vi "Get User Data.vi"(10 "USER/ITEM DATA TRANSFER":T1(array[cluster]), 11 "REFERENCES":T2) -> (2 "USER/ITEM DATA TRANSFER OUT":T1(array[cluster]), 3 "REFERENCES OUT":T2)   [LabVIEW 2019]
uses:
  Controls/References Cluster.ctl
  Controls/Custom Calendar/Custom Calendar.xctl
  Controls/Table Data Types/User Data Type.ctl
  <vilib>/vision/Image Controls.llb/IMAQ Image.ctl
  <vilib>/addons/database/Connection.llb/DB Tools Open Connec (String).vi
  <vilib>/addons/database/_DB Variant To Data/Database Variant To Data.xnode
  <vilib>/addons/database/NI_Database_API.lvlib
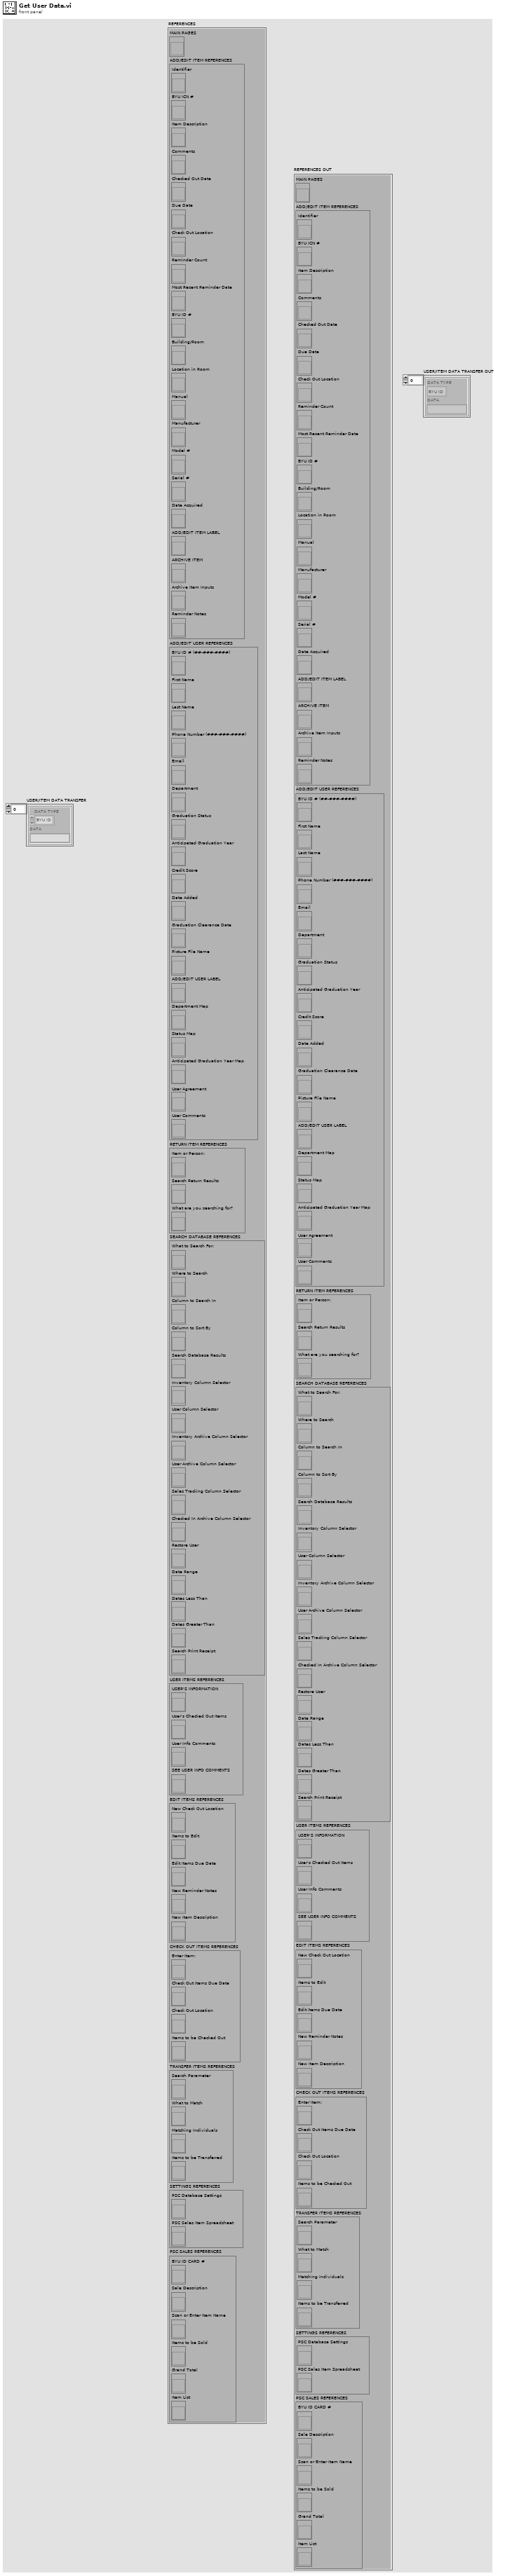
[diagram p1: front panel]
types:
  T1 = cluster{"DATA TYPE":enum16{"BYU ID", "ME#/IDENTIFIER", "BYU ICN"}, "DATA":string}[]
  T2 = typedef "References Cluster.ctl" = cluster{"MAIN PAGES":refnum<vi>, "ADD/EDIT ITEM REFERENCES":cluster{"Identifier":refnum<vi>, "BYU ICN #":refnum<vi>, "Item Description":refnum<vi>, "Comments":refnum<vi>, "Checked Out Date":refnum<vi>, "Due Date":refnum<vi>, "Check Out Location":refnum<vi>, "Reminder Count":refnum<vi>, "Most Recent Reminder Date":refnum<vi>, "BYU ID #":refnum<vi>, "Building/Room":refnum<vi>, "Location in Room":refnum<vi>, "Manual":refnum<vi>, "Manufacturer":refnum<vi>, "Model #":refnum<vi>, "Serial #":refnum<vi>, "Date Acquired":refnum<vi>, "ADD/EDIT ITEM LABEL":refnum<vi>, "ARCHIVE ITEM":refnum<vi>, "Archive Item Inputs":refnum<vi>, "Reminder Notes":refnum<vi>}, "ADD/EDIT USER REFERENCES":cluster{"BYU ID # (##-###-####)":refnum<vi>, "First Name":refnum<vi>, "Last Name":refnum<vi>, "Phone Number (###-###-####)":refnum<vi>, "Email":refnum<vi>, "Department":refnum<vi>, "Graduation Status":refnum<vi>, "Anticipated Graduation Year":refnum<vi>, "Credit Score":refnum<vi>, "Date Added":refnum<vi>, "Graduation Clearance Date":refnum<vi>, "Picture File Name":refnum<vi>, "ADD/EDIT USER LABEL":refnum<vi>, "Department Map":refnum<vi>, "Status Map":refnum<vi>, "Anticipated Graduation Year Map":refnum<vi>, "User Agreement":refnum<vi>, "User Comments":refnum<vi>}, "RETURN ITEM REFERENCES":cluster{"Item or Person:":refnum<vi>, "Search Return Results":refnum<vi>, "What are you searching for?":refnum<vi>}, "SEARCH DATABASE REFERENCES":cluster{"What to Search For:":refnum<vi>, "Where to Search":refnum<vi>, "Column to Search In":refnum<vi>, "Column to Sort By":refnum<vi>, "Search Database Results":refnum<vi>, "Inventory Column Selector":refnum<vi>, "User Column Selector":refnum<vi>, "Inventory Archive Column Selector":refnum<vi>, "User Archive Column Selector":refnum<vi>, "Sales Tracking Column Selector":refnum<vi>, "Checked In Archive Column Selector":refnum<vi>, "Restore User":refnum<vi>, "Date Range":refnum<vi>, "Dates Less Than":refnum<vi>, "Dates Greater Than":refnum<vi>, "Search Print Receipt":refnum<vi>}, "USER ITEMS REFERENCES":cluster{"USER'S INFORMATION":refnum<vi>, "User's Checked Out Items":refnum<vi>, "User Info Comments":refnum<vi>, "SEE USER INFO COMMENTS":refnum<vi>}, "EDIT ITEMS REFERENCES":cluster{"New Check Out Location":refnum<vi>, "Items to Edit":refnum<vi>, "Edit Items Due Date":refnum<vi>, "New Reminder Notes":refnum<vi>, "New Item Description":refnum<vi>}, "CHECK OUT ITEMS REFERENCES":cluster{"Enter Item:":refnum<vi>, "Check Out Items Due Date":refnum<vi>, "Check Out Location":refnum<vi>, "Items to be Checked Out":refnum<vi>}, "TRANSFER ITEMS REFERENCES":cluster{"Search Parameter":refnum<vi>, "What to Match":refnum<vi>, "Matching Individuals":refnum<vi>, "Items to be Transferred":refnum<vi>}, "SETTINGS REFERENCES":cluster{"PSC Database Settings":refnum<vi>, "PSC Sales Item Spreadsheet":refnum<vi>}, "PSC SALES REFERENCES":cluster{"BYU ID CARD #":refnum<vi>, "Sale Description":refnum<vi>, "Scan or Enter Item Name":refnum<vi>, "Items to be Sold":refnum<vi>, "Grand Total":refnum<vi>, "Item List":refnum<vi>}}
  T3 = enum32{"IDLE", "ADD/EDIT USER", "ADD/EDIT ITEM", "RETURN ITEMS", "SEARCH DATABASE", "USER ITEMS", "CHECK OUT ITEMS", "EDIT ITEMS", "TRANSFER ITEMS", "PSC SALES", "ATRIUM", "INVENTORY TRACKING", "SETTINGS"}
  T4 = typedef "IMAQ Image.ctl" = refnum<image>
  T5 = cluster{"BYU ID #":string, "First Name":string, "Last Name":string, "Phone Number":string, "Email":string, "Department":string, "Graduation Status":string, "Grad Year":string, "Credit Score":string, "Date Added":string, "Graduation Clearance Date":string, "User Items Photo":T4}
  T6 = typedef "User Data Type.ctl" = cluster{"BYU ID #":string, "First Name":string, "Last Name":string, "Phone Number":string, "Email":string, "Department":string, "Graduation Status":string, "Anticipated Graduation Year":string, "Credit Score":dbl, "Date Added":string, "Graduation Clearance Date":string, "Picture File Name":string, "User Comments":string}
  T7 = cluster{"DATA TYPE":enum16{"BYU ID", "ME#/IDENTIFIER", "BYU ICN"}, "DATA":string}
  T8 = typedef "NI_Database_API.lvlib/Conn ObjectReference.ctl" = refnum<k1>
  T9 = cluster{"USER'S INFORMATION":refnum<vi>, "User's Checked Out Items":refnum<vi>, "User Info Comments":refnum<vi>, "SEE USER INFO COMMENTS":refnum<vi>}
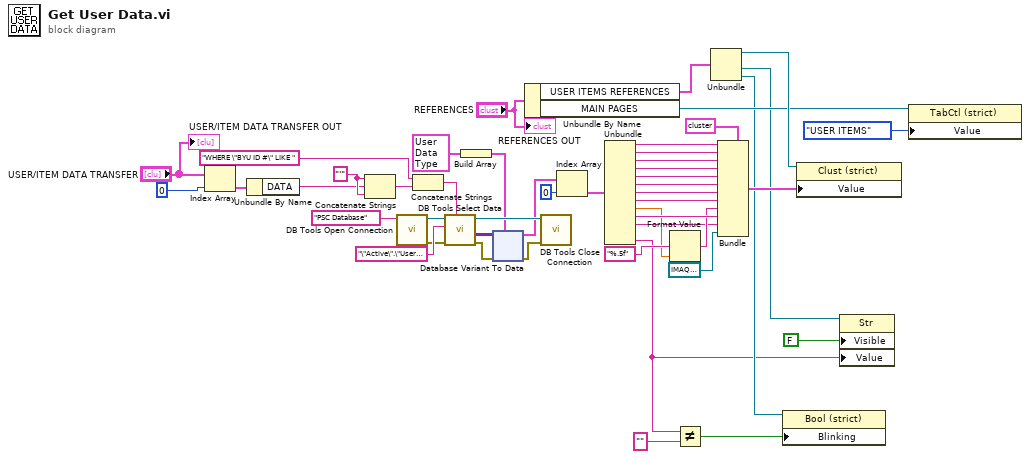
[diagram p0: block diagram]
diagram:
  w8 = "'" ("string")
  n1 = Index Array(array="USER/ITEM DATA TRANSFER", index=0) -> (element=w20:T7)
  n2 = Unbundle By Name(w20) -> ("DATA"=w7:string)
  n3 = Concatenate Strings(w8, w7, w8) -> (w9:string)
  n4 = call-poly <vilib>:"DB Tools Open Connection.vi"("connection information"="PSC Database") -> ("error out"=w45:errorcluster, "connection reference"=w46:T8)  [unwired: 7 in]
  n5 = Concatenate Strings("WHERE \"BYU ID #\" LIKE " ("string"), w9) -> (w43:string)
  n6 = call <vilib>:"DB Tools Select Data.vi"("condition"=w43, "error in (no error)"=w45, "table"="\"Active\".\"Users\"", "connection reference"=w46) -> ("error out"=w41:errorcluster, "data"=w42:variant[][], "connection reference out"=w40:T8)  [unwired: 2 in]
  n7 = Build Array(T6 {"BYU ID #"="", "First Name"="", "Last Name"="", "Phone Number"="", "Email"="", "Department"="", "Graduation Status"="", "Anticipated Graduation Year"="", "Credit Score"=0.0, "Date Added"="", "Graduation Clearance Date"="", "Picture File Name"="", "User Comments"=""} ("Array")) -> (w18:T6[])
  n8 = xnode "Database Variant To Data"("database variant"=w42, "error in (no error)"=w41, "type"=w18) -> ("data"=w38:T6[], "error out"=w39:errorcluster)
  n9 = Unbundle By Name("REFERENCES") -> ("USER ITEMS REFERENCES"=w23:T9, "MAIN PAGES"=w11:refnum<vi>)
  n10 = call <vilib>:"DB Tools Close Connection.vi"("error in (no error)"=w39, "connection reference"=w40) -> ()  [unwired: 5 in, 1 out]
  n11 = Index Array(array=w38, index=0) -> (element=w35:T6)
  n12 = Unbundle(w35) -> ("BYU ID #"=w34:string, "First Name"=w33:string, "Last Name"=w32:string, "Phone Number"=w31:string, "Email"=w30:string, "Department"=w29:string, "Graduation Status"=w28:string, "Anticipated Graduation Year"=w27:string, "Credit Score"=w17:dbl, "Date Added"=w26:string, "Graduation Clearance Date"=w14:string, "User Comments"=w1:string)  [unwired: 1 out]
  n13 = Format Value(format string="%.5f", value (0)=w17) -> (output string=w16:string)  [unwired: 1 in]
  n14 = Not Equal?(x=w1, y="") -> (x != y?=w2:bool)
  n15 = Unbundle(w23) -> ("USER'S INFORMATION"=w36:refnum<vi>, "User Info Comments"=w6:refnum<vi>, "SEE USER INFO COMMENTS"=w4:refnum<vi>)  [unwired: 1 out]
  n16 = Bundle(cluster=T5 {"BYU ID #"="", "First Name"="", "Last Name"="", "Phone Number"="", "Email"="", "Department"="", "Graduation Status"="", "Grad Year"="", "Credit Score"="", "Date Added"="", "Graduation Clearance Date"="", "User Items Photo"=refnum} ("USER'S INFORMATION"), "BYU ID #"=w34, "First Name"=w33, "Last Name"=w32, "Phone Number"=w31, "Email"=w30, "Department"=w29, "Graduation Status"=w28, "Grad Year"=w27, "Credit Score"=w16, "Date Added"=w26, "Graduation Clearance Date"=w14, "User Items Photo"=T4 refnum) -> (w12:T5)
  n17 = property class="Bool (strict)"(reference=w4, "Blinking"=w2) -> ()  [unwired: 1 in, 2 out]
  n18 = property class="Clust (strict)"(reference=w36, "Value"=w12) -> ()  [unwired: 1 in, 2 out]
  n19 = property class="Str"(reference=w6, "Visible"=FALSE, "Value"=w1) -> ()  [unwired: 1 in, 2 out]
  n20 = property class="TabCtl (strict)"(reference=w11, "Value"=T3."USER ITEMS") -> ()  [unwired: 1 in, 2 out]
  "REFERENCES OUT" <- "REFERENCES"
  "USER/ITEM DATA TRANSFER OUT" <- "USER/ITEM DATA TRANSFER"
